vi "test Connect Disconnect Multiple.vi"(8 "error in (no error)":errorcluster, 11 "TestCase in":refnum<class "%DEVICE% Messaging Tests.lvclass">) -> (0 "error out":errorcluster, 3 "TestCase out":refnum<class "%DEVICE% Messaging Tests.lvclass">)   [LabVIEW 2017, in "%DEVICE% Messaging Tests.lvclass"]
uses:
  %DEVICE% Messaging Tests.lvclass
  Includes/CDMessaging.lvlibp/Switch/Switch Disconnect Message/Switch Disconnect Message.lvclass
  C:/Users/Admin/Documents/niveristand-routing-and-faulting-message-library/Includes/CDMessaging.lvlibp/Message/Abstract Message/Abstract Message.lvclass
  Includes/CDMessaging.lvlibp/Switch/Switch Connect Message/Switch Connect Message.lvclass
  Support/Mock %DEVICE% Consumer.lvclass
  %DEVICE% Messaging Tests.lvclass/%DEVICE% Messaging Tests.ctl
  Support/Mock %DEVICE% Consumer.lvclass/Mock %DEVICE% Consumer.ctl
  Support/Read Connections.vi
  Includes/CDMessaging.lvlibp/Switch/Abstract Switch Consumer/Abstract Switch Consumer.lvclass
  C:/Users/Admin/Documents/niveristand-routing-and-faulting-message-library/Includes/CDMessaging.lvlibp/Consumer/Abstract Consumer/Abstract Consumer.lvclass
  Includes/CDMessaging.lvlibp/Producer/Abstract Producer/Abstract Producer.lvclass
  <vilib>/addons/_JKI Toolkits/VI Tester/TestCase.llb/TestCase.lvclass
  Includes/CDMessaging.lvlibp/Consumer/Abstract Consumer/Abstract Consumer.lvclass
  C:/Program Files (x86)/National Instruments/LabVIEW 2017/vi.lib/addons/_JKI Toolkits/VI Tester/TestCase.llb/TestCase.lvclass
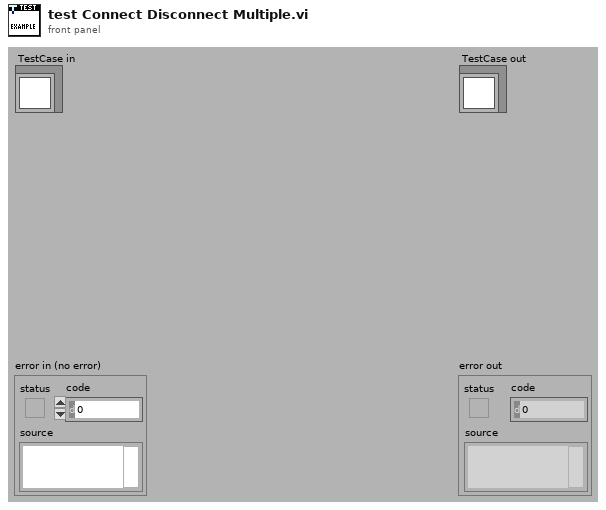
[diagram p1: front panel]
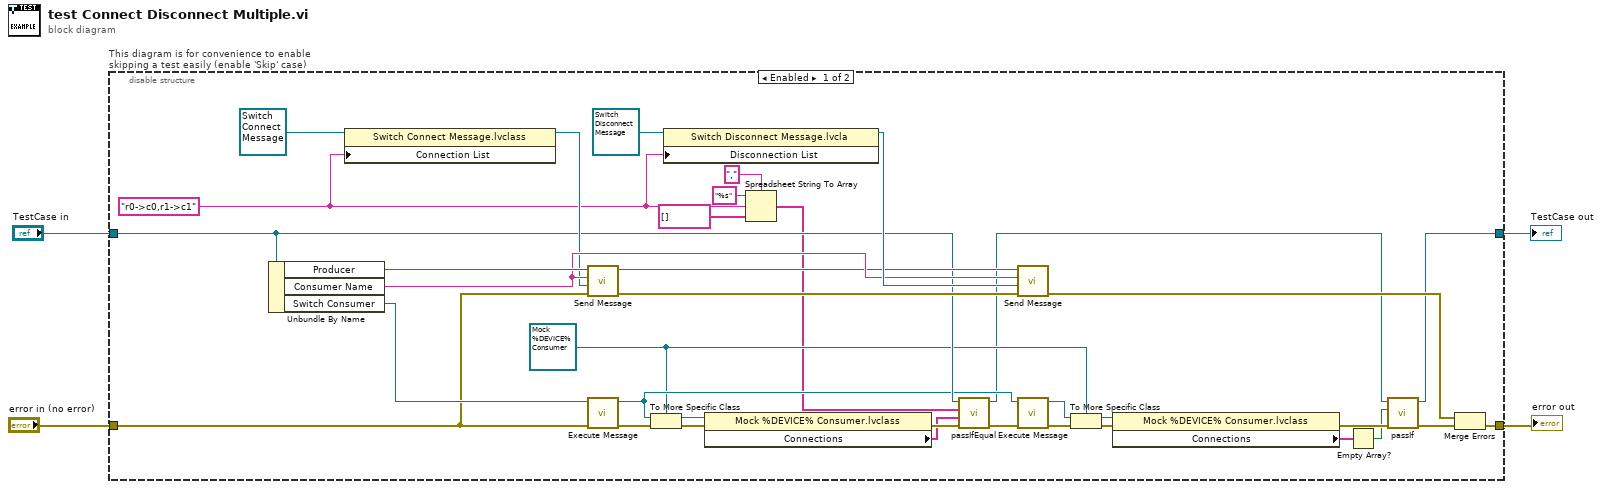
[diagram p0: block diagram]
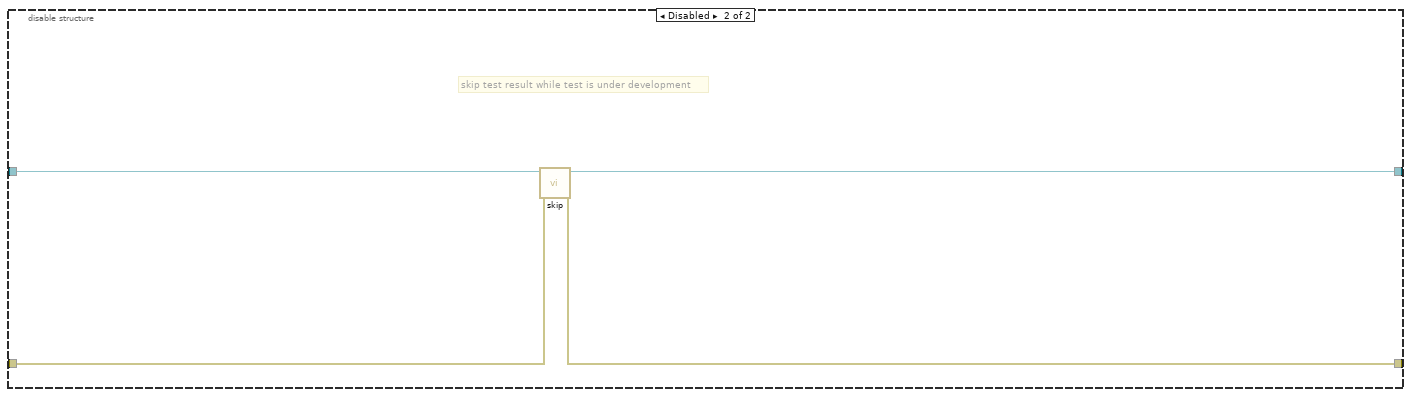
[diagram p2: hidden frame]
diagram:
  n1 = disable-structure "This diagram is for convenience to enable skipping a test easily (enable 'Skip' case)" shown="Enabled" {
    disable-tunnel: "TestCase in" -> [w22 w44]
    disable-tunnel: [w13 w42] -> w1
    disable-tunnel: [w36 w43] -> w3
    disable-tunnel: "error in (no error)" -> [w33 w41]
    frame Enabled {
      w17 = refnum<class "Mock %DEVICE% Consumer.lvclass"> refnum ("Mock NI-SWITCH Consumer.lvclass")
      w9 = "r0->c0,r1->c1"
      n2 = Unbundle By Name(w22) -> ("Producer"=w35:refnum<class "Abstract Producer.lvclass">, "Consumer Name"=w34:string, "Switch Consumer"=w38:refnum<class "Abstract Switch Consumer.lvclass">)
      n3 = property class="Switch Connect Message.lvclass"(reference=refnum<class "Switch Connect Message.lvclass"> refnum ("CDMessaging.lvlibp:Switch Connect Message.lvclass"), "Connection List"=w9) -> (reference out=w29:refnum<class "Switch Connect Message.lvclass">)  [unwired: 1 in, 1 out]
      n4 = call-dynamic "Send Message.vi"("error in (no error)"=w33, "Message in"=w29, "Consumer in"=w34, "Abstract Producer in"=w35) -> ("error out"=w32:errorcluster, "Abstract Producer out"=w31:refnum<class "Abstract Producer.lvclass">)  [unwired: 4 in, 2 out]
      n5 = call "Execute Message.vi"("error in (no error)"=w33, "Abstract Consumer in"=w38) -> ("error out"=w28:errorcluster, "Abstract Consumer out"=w21:refnum<class "Abstract Consumer.lvclass">)  [unwired: 6 in, 2 out]
      n6 = To More Specific Class(target class=w17, reference=w21, error in=w28) -> (specific class reference=w26:refnum<class "Mock %DEVICE% Consumer.lvclass">, error out=w27:errorcluster)
      n7 = property class="Switch Disconnect Message.lvcla"(reference=refnum<class "Switch Disconnect Message.lvclass"> refnum ("CDMessaging.lvlibp:Switch Disconnect Message.lvclass"), "Disconnection List"=w9) -> (reference out=w39:refnum<class "Switch Disconnect Message.lvclass">)  [unwired: 1 in, 1 out]
      n8 = property class="Mock %DEVICE% Consumer.lvclass"(reference=w26, error in=w27) -> (error out=w25:errorcluster, "Connections"=w24:string[])  [unwired: 1 out]
      n9 = Spreadsheet String To Array(delimiter (Tab)=",", format string="%s", spreadsheet string=w9, array type (2D Dbl)=string[] []) -> (array=w8:string[])
      n10 = call-dynamic "passIfEqual.vi"("error in (no error)"=w25, "y"=w24, "x"=w8, "TestCase in"=w22) -> ("error out"=w23:errorcluster, "TestCase out"=w14:refnum<class "%DEVICE% Messaging Tests.lvclass">)  [unwired: 6 in]
      n11 = call-dynamic "Send Message.vi"("error in (no error)"=w32, "Message in"=w39, "Consumer in"=w34, "Abstract Producer in"=w31) -> ("error out"=w37:errorcluster)  [unwired: 4 in, 3 out]
      n12 = call "Execute Message.vi"("error in (no error)"=w23, "Abstract Consumer in"=w21) -> ("error out"=w19:errorcluster, "Abstract Consumer out"=w18:refnum<class "Abstract Consumer.lvclass">)  [unwired: 6 in, 2 out]
      n13 = To More Specific Class(target class=w17, reference=w18, error in=w19) -> (specific class reference=w12:refnum<class "Mock %DEVICE% Consumer.lvclass">, error out=w20:errorcluster)
      n14 = property class="Mock %DEVICE% Consumer.lvclass"(reference=w12, error in=w20) -> (error out=w16:errorcluster, "Connections"=w11:string[])  [unwired: 1 out]
      n15 = Empty Array?(array=w11) -> (empty?=w10:bool)
      n16 = call-dynamic "passIf.vi"("error in (no error)"=w16, "pass"=w10, "TestCase in"=w14) -> ("error out"=w15:errorcluster, "TestCase out"=w13:refnum<class "%DEVICE% Messaging Tests.lvclass">)  [unwired: 7 in]
      n17 = Merge Errors(w37, w15) -> (w36:errorcluster)
    }
    frame Disabled {
      # "skip test result while test is under development"
      n18 = call <vilib>:"skip.vi"("error in (no error)"=w41, "TestCase in"=w44) -> ("error out"=w43:errorcluster, "TestCase out"=w42:refnum<class "%DEVICE% Messaging Tests.lvclass">)  [unwired: 8 in]
    }
  }
  "error out" <- w3
  "TestCase out" <- w1
